vi "Analyze Coefficients-Quantized Filter.vi"() -> ()   [LabVIEW 2023]
doc: "Demonstrates how to use the DFD FXP Coef Report VI and the Filter Analysis VIs to analyze a quantized filter.\n\nComplete the following steps to use this VI.\n1) Design a filter by setting the specifications.\n2) Run the VI.\n3) Observe both the floating-point and fixed-point filter responses, such as the magnitude response, phase response, group delay, and others.\n4) Observe the Coefficients Report to compare the Quantized Value with the Reference Value.\n5) Change the <B>Coefficients a/k Word Length</B> and <B>Coefficients b/v Word Length</B> values. Refer to the LabVIEW Help for more information about the coefficients a/k and coefficients b/v.\n6) Change the <B>Gain Settings</B> to specify whether to process the filter gain on a host machine or a fixed-point target.\n7) Run the VI again.\n8) Observe the fixed-point and floating-point filter responses and determine whether overflow, underflow, or zeroes occurred during the coefficient quantization.\n9) Observe the Coefficients Quantizers to understand what the actual coefficients quantizer settings are.\n10) Observe the Coefficients Report to understand how this VI processes the filter gain.\n\n<B>Note:</B> Examine the Pole-Zero plot to determine if the filter is stable after coefficients quantization."
uses:
  <vilib>/addons/Digital Filter Design/_Objects.llb/DFD Filter Frequence Specification (Design).ctl
  <vilib>/addons/Digital Filter Design/_Objects.llb/DFD Pole-Zero Plot.ctl
  <vilib>/addons/Digital Filter Design/_Objects.llb/DFD Quantization Settings.ctl
  <vilib>/addons/Digital Filter Design/_Objects.llb/DFD Quantization Sources.ctl
  <vilib>/addons/Digital Filter Design/_Objects.llb/DFD Phase Setting.ctl
  <vilib>/addons/Digital Filter Design/FXPModel.llb/DFD FXP Quantize Coef (Easy).vi
  <vilib>/addons/Digital Filter Design/Analysis.llb/DFD Plot Freq Response (Linear-Spaced).vi
  <vilib>/addons/Digital Filter Design/FXPModel.llb/DFD FXP Get Quantizer (Group).vi
  <vilib>/addons/Digital Filter Design/NI_DigFilterLicensed.lvlib
panel:
  out "Coefficients Quantizers":T1[](array[typedef]) {"source" items=["Coefficients a/k"=0, "Coefficients b/v"=7, "Input"=1, "Output"=2, "Multiplicand"=3, "Product"=4, "Sum"=5, "Delay"=6]}
  in  "Gain Settings":T3={"gain processing"=1, "gain word length"=16} {"gain processing" items=["On Target", "On Host"]}
  in  "Coefficients b/v Word Length":i16=16
  in  "Coefficients a/k Word Length":i16=16
  out "Error Message":string
  in  "Design Method":T4(ring)=enum."Chebyshev"
  in  "Sampling Frequency [Hz]":dbl=1000.0 format="%.2f"
  in  "Analysis Tab":T5(tab)
  out "Magnitude Response":cluster{"f0":dbl, "df":dbl, "values":dbl[]}[](graph)
  out "Phase Response":cluster{"f0":dbl, "df":dbl, "values":dbl[]}[](graph)
  out "Group Delay":cluster{"f0":dbl, "df":dbl, "values":dbl[]}[](graph)
  out "Z-Plane":T6
  out "Impulse Response":T7(graph)
  out "Step Response":T7(graph)
  in  "Filter Type":u16(ring)=2 items=["Lowpass", "Highpass", "Bandpass", "Bandstop"]
  out "Coefficients Report":string
  in  "Frequency Sepcifications [Hz]":T8={"fpass 1"=200.0, "fstop 1"=100.0, "fpass 2 "=300.0, "fstop 2"=400.0}
  # "Select Help>>Show Context Help and move the cursor over the VI icon for more information."
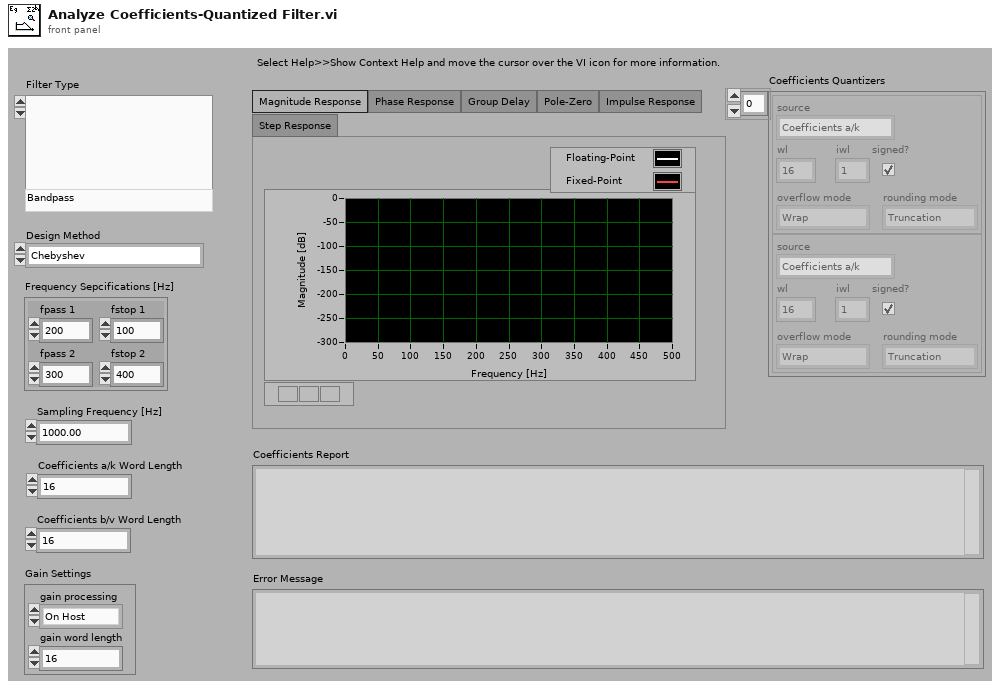
[diagram p1: front panel]
types:
  T1 = typedef "NI_DigFilterLicensed.lvlib/DFD Quantization Settings.ctl" = cluster{"source":T2, "wl":i16, "iwl":i16, "overflow mode":enum16{"Saturation", "Wrap"}, "rounding mode":enum16{"Nearest", "Truncation"}, "signed?":bool}
  T2 = typedef "NI_DigFilterLicensed.lvlib/DFD Quantization Sources.ctl" = u16
  T3 = cluster{"gain processing":u16, "gain word length":i16}
  T4 = enum16{"Butterworth", "Chebyshev", "Inverse Chebyshev", "Elliptic", "Kaiser Window", "Dolph-Chebyshev Window", "Equi-Ripple FIR"}
  T5 = enum32{"Magnitude Response", "Phase Response", "Group Delay", "Pole-Zero", "Impulse Response", "Step Response"}
  T6 = typedef "NI_DigFilterLicensed.lvlib/DFD Pole-Zero Plot.ctl" = cluster{dbl[], dbl[]}[]
  T7 = cluster{"t0":dbl, "dt":dbl, "amplitudes":dbl[]}[]
  T8 = typedef "NI_DigFilterLicensed.lvlib/DFD Filter Frequence Specification (Design).ctl" = cluster{"fpass 1":dbl, "fstop 1":dbl, "fpass 2 ":dbl, "fstop 2":dbl}
  T9 = typedef "NI_DigFilterLicensed.lvlib/DFD Phase Setting.ctl" = cluster{"unwrap? (F)":bool, "degree? (F)":bool}
  T10 = typedef "NI_DigFilterLicensed.lvlib/DFD Filter Obj.ctl" = cluster{"mSRate_Fs":dbl, "mSRate_Version":string, "mSRate_Comments":string, "mSRate_OrgCoef":T11, "mSRate_CurCoef":T11, "mSRate_Quantized?":bool, "mSRate_QCoef":T11, "mSRate_QSettings":T13[], "mSRate_Order":i32, "mSRate_Scaling":cluster{"mSRate_ScaleByPowerOf2?":bool, "mSRate_ScaleType":T15}}
  T11 = typedef "NI_DigFilterLicensed.lvlib/DFD Filter Coef.ctl" = cluster{"type":T12, "gain":dbl, "coef a (k)":dbl[], "coef b (v)":dbl[]}
  T12 = typedef "NI_DigFilterLicensed.lvlib/DFD Filter Structure Type Selector.ctl" = enum16{"Undefined", "FIR Direct Form", "FIR Direct Form Transposed", "FIR Symmetric", "FIR Antisymmetric", "IIR Direct Form I", "IIR Direct Form I Transposed", "IIR Direct Form II", "IIR Direct Form II Transposed", "IIR Cascaded Second Order Sections Form I", "IIR Cascaded Second Order Sections Form I Transposed", "IIR Cascaded Second Order Sections Form II", "IIR Cascaded Second Order Sections Form II Transposed", "Lattice Allpass (basic sections)", "Lattice Allpass (one multiplier sections)", "Lattice Allpass (normalized sections)", "Lattice AR (basic sections)", "Lattice AR (one multiplier sections)", "Lattice AR (normalized sections)", "Lattice MA (minimum phase)", "Lattice MA (maximum phase)", "Lattice ARMA (basic sections)", "Lattice ARMA (one multiplier sections)", "Lattice ARMA (normalized sections)"}
  T13 = typedef "NI_DigFilterLicensed.lvlib/dfd_Internal Quantization Settings.ctl" = cluster{"source":T14, "wl":i16, "iwl":i16, "overflow mode":enum16{"Saturation", "Wrap"}, "rounding mode":enum16{"Nearest", "Truncation"}, "signed?":bool}
  T14 = typedef "NI_DigFilterLicensed.lvlib/dfd_Internal Quantization Srcs.ctl" = u16
  T15 = typedef "NI_DigFilterLicensed.lvlib/DFD Coef Norm Type.ctl" = enum16{"No Norm", "Time Domain 1-Norm", "Time Domain 2-Norm", "Time Domain Inf-Norm"}
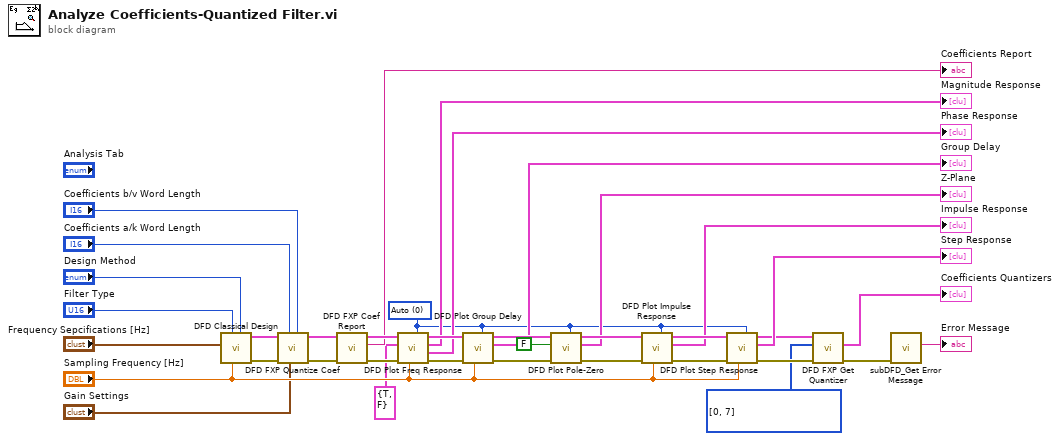
[diagram p0: block diagram]
diagram:
  w2 = T2[] [0, 7] items=["Coefficients a/k"=0, "Coefficients b/v"=7, "Input"=1, "Output"=2, "Multiplicand"=3, "Product"=4, "Sum"=5, "Delay"=6] ("quantizer sources")
  w14 = u16 0 items=["Auto", "Floating-point Only", "Fixed-point Only"] ("output option")
  n1 = call <vilib>:"DFD Classical Design.vi"("design method"="Design Method", "fs [Hz]"="Sampling Frequency [Hz]", "filter type"="Filter Type", "freq specs [Hz]"="Frequency Sepcifications [Hz]") -> ("error out"=w35:errorcluster, "filter out"=w36:T10)  [unwired: 2 in, 4 out]
  n2 = call-poly <vilib>:"DFD FXP Quantize Coef.vi"("coefficients b/v word length"="Coefficients b/v Word Length", "gain settings"="Gain Settings", "coefficients a/k word length"="Coefficients a/k Word Length", "error in (no error)"=w35, "filter in"=w36) -> ("error out"=w24:errorcluster, "filter out"=w26:T10)  [unwired: 5 out]
  n3 = call <vilib>:"DFD FXP Coef Report.vi"("error in (no error)"=w24, "filter in"=w26) -> ("error out"=w23:errorcluster, "coefficients report"=→"Coefficients Report":string, "filter out"=w25:T10)  [unwired: 7 out]
  n4 = call-poly <vilib>:"DFD Plot Freq Response.vi"("output option"=w14, "fs [Hz]"="Sampling Frequency [Hz]", "error in (no error)"=w23, "phase view"=T9 {"unwrap? (F)"=TRUE, "degree? (F)"=FALSE}, "filter in"=w25) -> ("error out"=w33:errorcluster, "phase response"=→"Phase Response":cluster{"f0":dbl, "df":dbl, "values":dbl[]}[], "magnitude response"=→"Magnitude Response":cluster{"f0":dbl, "df":dbl, "values":dbl[]}[], "filter out"=w34:T10)  [unwired: 3 in]
  n5 = call <vilib>:"DFD Plot Group Delay.vi"("output option"=w14, "fs [Hz]"="Sampling Frequency [Hz]", "error in (no error)"=w33, "filter in"=w34) -> ("error out"=w31:errorcluster, "group delay"=→"Group Delay":cluster{"f0":dbl, "df":dbl, "values":dbl[]}[], "filter out"=w32:T10)  [unwired: 1 in, 4 out]
  n6 = call <vilib>:"DFD Plot Pole-Zero.vi"("output option"=w14, "error in (no error)"=w31, "upper half plane only"=FALSE, "filter in"=w32) -> ("error out"=w29:errorcluster, "Z-Plane"=→"Z-Plane":T6, "filter out"=w30:T10)  [unwired: 5 out]
  n7 = call <vilib>:"DFD Plot Impulse Response.vi"("output option"=w14, "fs [Hz]"="Sampling Frequency [Hz]", "error in (no error)"=w29, "filter in"=w30) -> ("error out"=w27:errorcluster, "impulse response"=→"Impulse Response":T7, "filter out"=w28:T10)  [unwired: 1 in, 4 out]
  n8 = call <vilib>:"DFD Plot Step Response.vi"("output option"=w14, "fs [Hz]"="Sampling Frequency [Hz]", "error in (no error)"=w27, "filter in"=w28) -> ("error out"=w5:errorcluster, "step response"=→"Step Response":T7, "filter out"=w3:T10)  [unwired: 1 in, 4 out]
  n9 = call-poly <vilib>:"DFD FXP Get Quantizer.vi"("error in (no error)"=w5, "quantizer sources"=w2, "filter in"=w3) -> ("error out"=w4:errorcluster, "quantizers"=→"Coefficients Quantizers":T1[])  [unwired: 7 out]
  n10 = call <vilib>:"subDFD_Get Error Message.vi"("error in (no error)"=w4) -> ("Error Message"=→"Error Message":string)  [unwired: 10 out]
